vi "I2C Grove TrackerEyeballs.vi"() -> ()   [LabVIEW 2020, in "CTI-Scratchpad.lvlib"]
uses:
  CTI-Scratchpad.lvlib
  CTI/Identity.ctl
  CTI/Error Reporting.ctl
  CTI/GPIO Number.ctl
  CTI/I2C Number.ctl
  CTI/Session/Session.lvclass
  CTI-Peripheral/I2C OLED/48x64 I2C OLED SSD1306/48x64 I2C OLED SSD1306.lvclass
  CTI-Peripheral/Thermal Camera/I2C Thermal Camera/AMG8833 8x8/AMG8833 8x8 Camera.lvclass
  CTI/VisaComms/VisaComms.lvclass
  CTI/CTI.lvlib
panel:
  out "max index(es)":i32[](array[numeric])
  out "Intensity Graph 2":dbl[][](graph)
  out "2D Picture 2":picture
  out "Identity":T1
  in  "stop":bool
  out "2D Picture":picture
  out "error out":errorcluster
  in  "Port":refnum<visa-resource-name>="COM4"
  # "https://wiki.seeedstudio.com/Grove-OLED-Display-0.66-SSD1306_v1.0/"
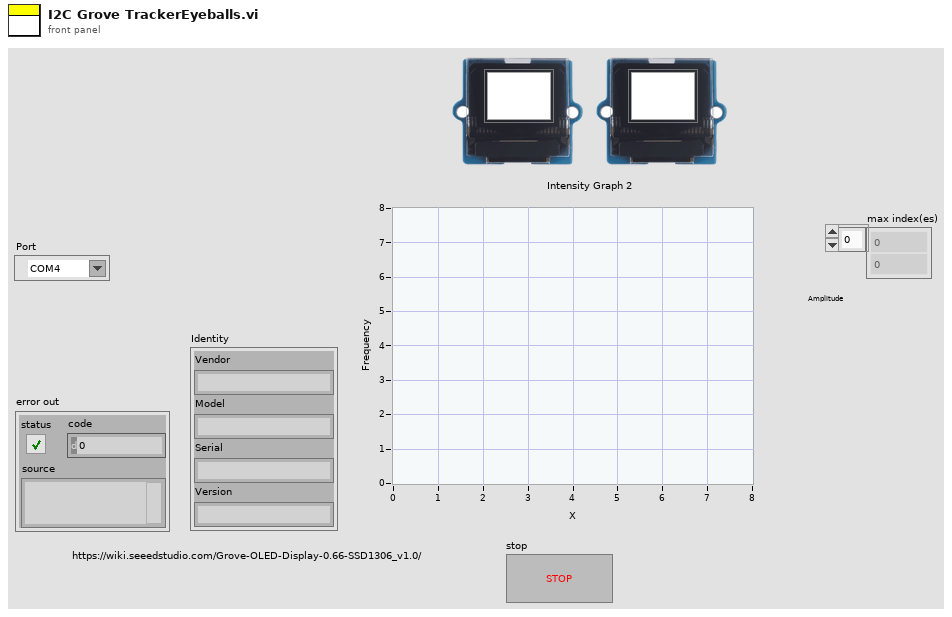
[diagram p1: front panel]
types:
  T1 = typedef "CTI.lvlib/Identity.ctl" = cluster{"Vendor":string, "Model":string, "Serial":string, "Version":string}
  T2 = typedef "CTI.lvlib/I2C Number.ctl" = i8
  T3 = typedef "CTI.lvlib/GPIO Number.ctl" = i8
  T4 = typedef "CTI.lvlib/Error Reporting.ctl" = enum16{"Minimal", "Moderate", "Full"}
  T5 = typedef "imagedata.ctl" = cluster{"image type":i32, "image depth":i32, "image":u8[], "mask":u8[], "colors":u32[], "Rectangle":cluster{"left":i16, "top":i16, "right":i16, "bottom":i16}}
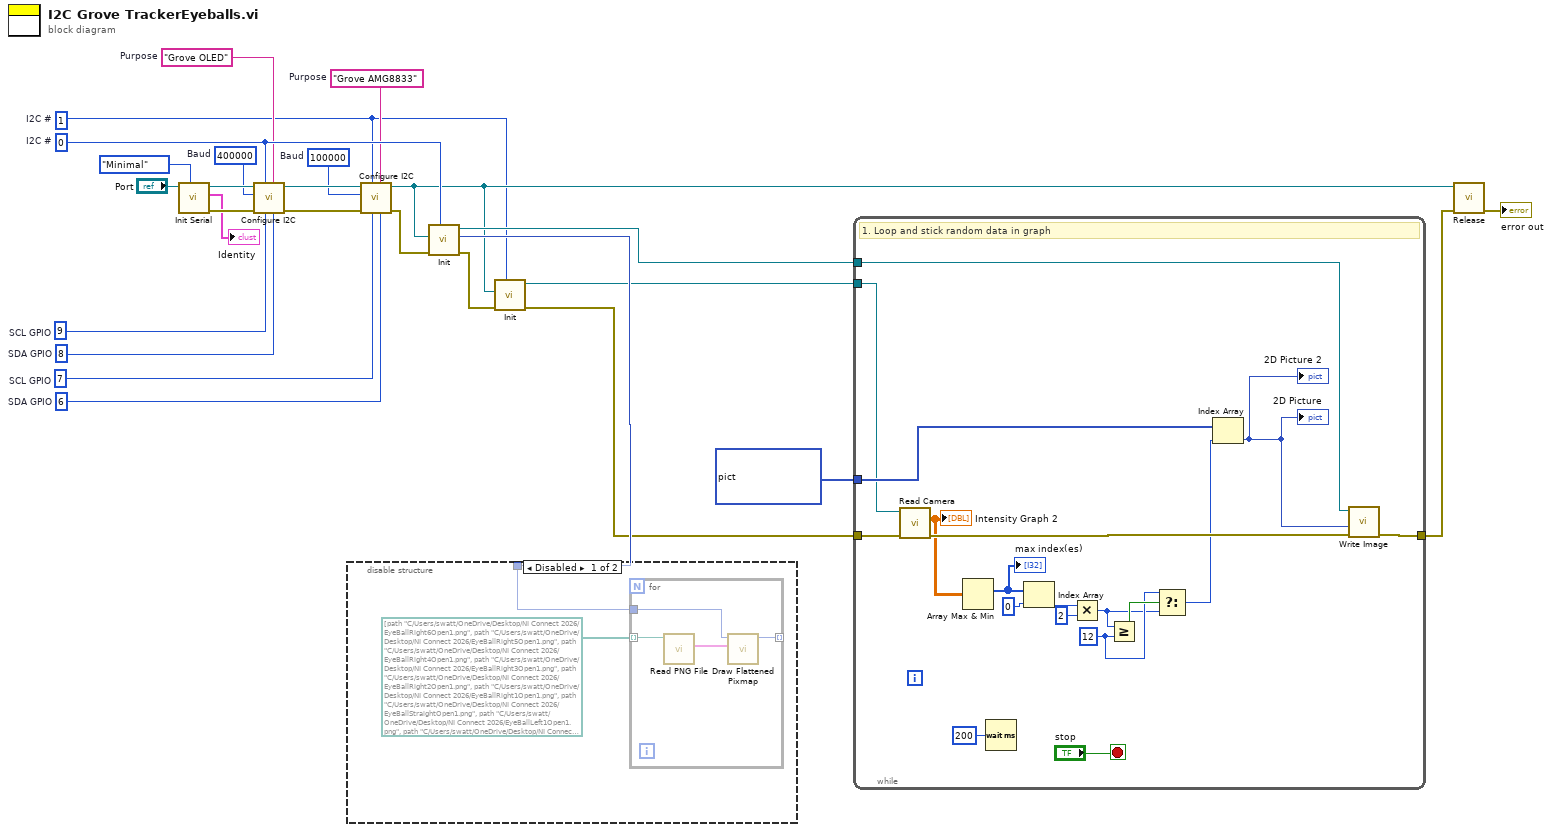
[diagram p0: block diagram]
diagram:
  w6 = "Grove AMG8833"  # Purpose
  w9 = u32 100000  # Baud
  w21 = T2 0  # I2C #
  w22 = T3 8  # SDA GPIO
  w23 = T3 9  # SCL GPIO
  w4 = T2 1  # I2C #
  w7 = T3 6  # SDA GPIO
  w8 = T3 7  # SCL GPIO
  w16 = "Grove OLED"  # Purpose
  w10 = u32 400000  # Baud
  n1 = call "Init Serial.vi"("Error Checking (Full)"=Error_Reporting."Minimal", "VISA resource name in"="Port") -> ("error out"=w24:errorcluster, "Identity"=→"Identity":T1, "Session"=w25:refnum<class "Session.lvclass">)  [unwired: 7 in]
  n2 = call "Configure I2C.vi"("SDA GPIO"=w22, "Purpose (\"I2C\")"=w16, "SCL GPIO"=w23, "I2C #"=w21, "error in (no error)"=w24, "Baud"=w10, "Session in"=w25) -> ("error out"=w13:errorcluster, "Session out"=w12:refnum<class "Session.lvclass">)  [unwired: 3 in]
  n3 = call "Configure I2C.vi"("SDA GPIO"=w7, "Purpose (\"I2C\")"=w6, "SCL GPIO"=w8, "I2C #"=w4, "error in (no error)"=w13, "Baud"=w9, "Session in"=w12) -> ("error out"=w11:errorcluster, "Session out"=w5:refnum<class "Session.lvclass">)  [unwired: 3 in]
  n4 = call "Init.vi"("I2C #"=w21, "error in (no error)"=w11, "Session In"=w5) -> ("error out"=w3:errorcluster, "2D Picture"=w15:picture, "48x64 I2C OLED SSD1306 Out"=w19:refnum<class "48x64 I2C OLED SSD1306.lvclass">)  [unwired: 6 in]
  n5 = disable-structure shown="Disabled" {
    disable-tunnel: w15 -> [w29 _]
    frame Disabled {
      n6 = for {
        tunnel: [w33] -> _ mode=indexing
        tunnel: w29 -> [w32]
        tunnel: path[] [path "C:/Users/swatt/OneDrive/Desktop/NI Connect 2026/EyeBallRight6Open1.png", path "C:/Users/swatt/OneDrive/Desktop/NI Connect 2026/EyeBallRight5Open1.png", path "C:/Users/swatt/OneDrive/Desktop/NI Connect 2026/EyeBallRight4Open1.png", path "C:/Users/swatt/OneDrive/Desktop/NI Connect 2026/EyeBallRight3Open1.png", path "C:/Users/swatt/OneDrive/Desktop/NI Connect 2026/EyeBallRight2Open1.png", path "C:/Users/swatt/OneDrive/Desktop/NI Connect 2026/EyeBallRight1Open1.png", path "C:/Users/swatt/OneDrive/Desktop/NI Connect 2026/EyeBallStraightOpen1.png", path "C:/Users/swatt/OneDrive/Desktop/NI Connect 2026/EyeBallLeft1Open1.png", path "C:/Users/swatt/OneDrive/Desktop/NI Connect 2026/EyeBallLeft2Open1.png", path "C:/Users/swatt/OneDrive/Desktop/NI Connect 2026/EyeBallLeft3Open1.png", path "C:/Users/swatt/OneDrive/Desktop/NI Connect 2026/EyeBallLeft4Open1.png", path "C:/Users/swatt/OneDrive/Desktop/NI Connect 2026/EyeBallLeft5Open1.png", path "C:/Users/swatt/OneDrive/Desktop/NI Connect 2026/EyeBallLeft6Open1.png"] -> [w31] mode=indexing
        n7 = call <vilib>:"Read PNG File.vi"("path to PNG file"=w31) -> ("image data"=w30:T5)  [unwired: 8 in, 2 out]
        n8 = call <vilib>:"Draw Flattened Pixmap.vi"("image data"=w30, "picture"=w32) -> ("new picture"=w33:picture)  [unwired: 7 in]
      }
    }
    frame Enabled {
    }
  }
  n9 = call "Init.vi"("I2C #"=w4, "error in (no error)"=w3, "Session In"=w5) -> ("error out"=w2:errorcluster, "AMG8833 8x8 Camera Out"=w1:refnum<class "AMG8833 8x8 Camera.lvclass">)  [unwired: 7 in]
  n10 = while {
    tunnel: w2 -> [w45]
    tunnel: w19 -> [w47]
    tunnel: [w46] -> w18
    tunnel: picture[] [bytes[5152], bytes[5152], bytes[5152], bytes[5152], bytes[5152], bytes[5152], bytes[5152], bytes[5152], bytes[5152], bytes[5152], bytes[5152], bytes[5152], bytes[5152]] ("Array") -> [w49]
    tunnel: w1 -> [w44]
    stop <- "stop" stop-if-true
    w36 = 12 ("y")
    # "1. Loop and stick random data in graph"
    n11 = call-dynamic "Read Camera.vi"("error in (no error)"=w45, "AMG8833 8x8 Camera in"=w44) -> ("error out"=w43:errorcluster, "Camera Output"=w42:dbl[][])  [unwired: 7 in, 1 out]
    "Intensity Graph 2" <- w42
    n12 = Array Max & Min(array=w42) -> (max index (indices)=w41:i32[])  [unwired: 3 out]
    "max index(es)" <- w41
    n13 = Wait (ms)(milliseconds to wait=u32 200) -> ()  [unwired: 1 out]
    n14 = Index Array(array=w41, index=0) -> (element=w39:i32)
    n15 = Multiply(x=w39, y=2) -> (x*y=w35:i32)
    n16 = Greater Or Equal?(x=w35, y=w36) -> (x >= y?=w37:bool)
    n17 = Select(t=w36, s=w37, f=w35) -> (s? t:f=w34:i32)
    n18 = Index Array(array=w49, index=w34) -> (element=w48:picture)
    "2D Picture" <- w48
    "2D Picture 2" <- w48
    n19 = call-dynamic "Write Image.vi"("error in (no error)"=w43, "2D Picture"=w48, "48x64 I2C OLED SSD1306 In"=w47) -> ("error out"=w46:errorcluster)  [unwired: 7 in, 1 out]
  }
  n20 = call-dynamic "Release.vi"("error in (no error)"=w18, "Session in"=w5) -> ("error out"=→"error out":errorcluster)  [unwired: 9 in]
